vi "Serial Write to DB.vi"(8 "error in":errorcluster, 9 "Chamber ID":T2(array[cluster])=[{"Chamber name"="Analysis", "Trip pressure"=5e-07}, {"Chamber name"="Prep", "Trip pressure"=3e-05}], 10 "AML Cluster const":T1[](array[typedef]), 11 "Data.PG in":refnum<class "LV-Data.PGSQL.lvclass">) -> (0 "error out":errorcluster, 1 "Paths":string[](array[string]), 2 "Successful Writes":bool[](array[boolean]), 3 "Data.PG out":refnum<class "LV-Data.PGSQL.lvclass">)   [LabVIEW 2019, in "PGC2D.lvlib"]
uses:
  PGC2D.lvlib
  <userlib>/LevyLab/LV-Data/LV-Data.PG/LV-Data.PGSQL.lvclass
  sandbox/Instrument.AML.GetAll--Cluster.ctl
  <userlib>/LevyLab/LV-Data/LV-Data.PG/API/Write Variable (one-row).vi
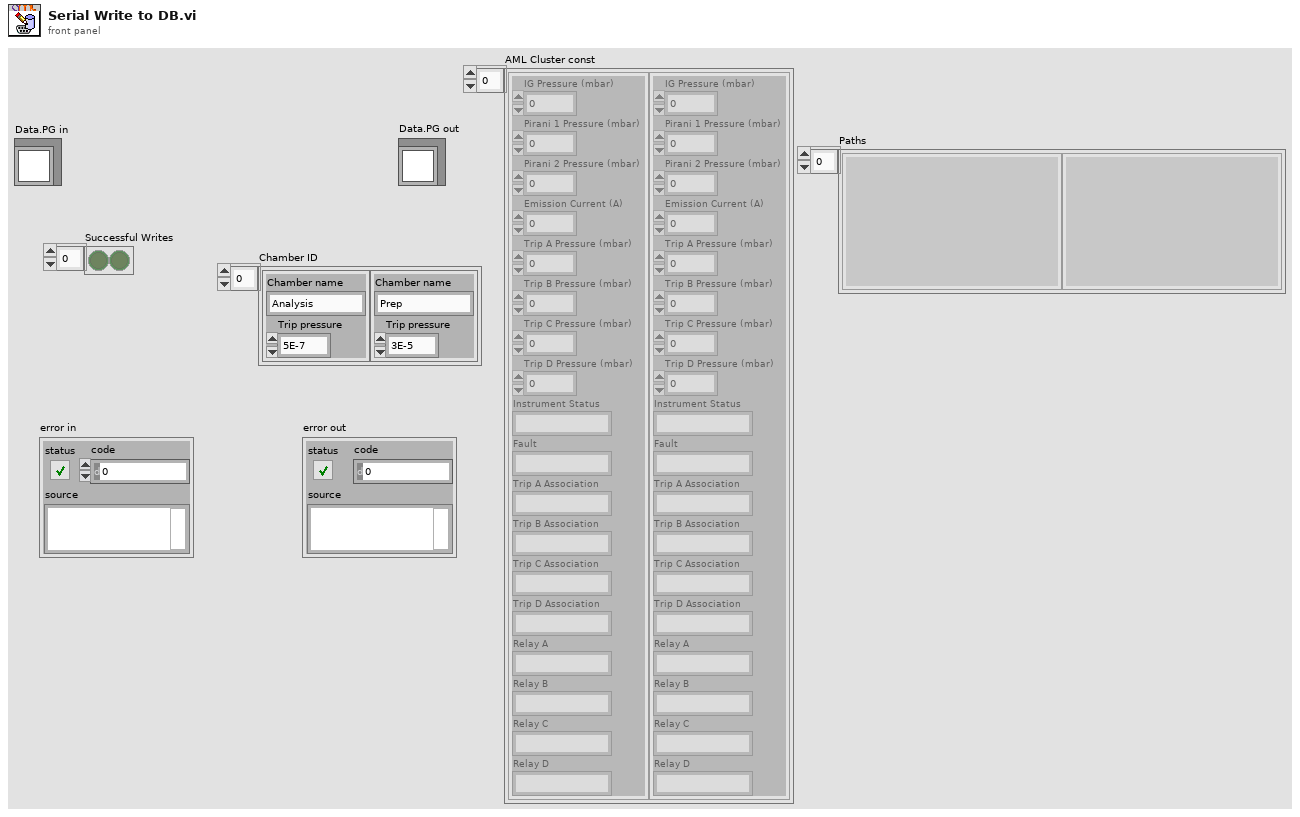
[diagram p1: front panel]
types:
  T1 = typedef "Instrument.AML.GetAll--Cluster.ctl" = cluster{"IG Pressure (mbar)":dbl, "Pirani 1 Pressure (mbar)":dbl, "Pirani 2 Pressure (mbar)":dbl, "Emission Current (A)":dbl, "Trip A Pressure (mbar)":dbl, "Trip B Pressure (mbar)":dbl, "Trip C Pressure (mbar)":dbl, "Trip D Pressure (mbar)":dbl, "Instrument Status":string, "Fault":string, "Trip A Association":string, "Trip B Association":string, "Trip C Association":string, "Trip D Association":string, "Relay A":string, "Relay B":string, "Relay C":string, "Relay D":string}
  T2 = cluster{"Chamber name":string, "Trip pressure":dbl}[]
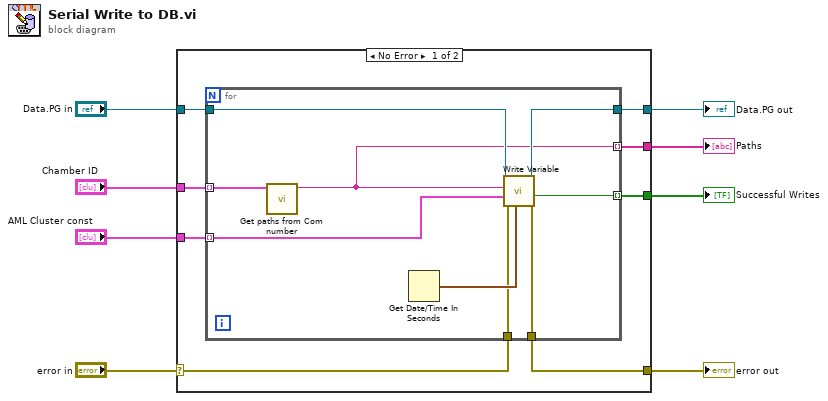
[diagram p0: block diagram]
diagram:
  n1 = case shown="No Error" "error in" {
    selector: "error in" -> [w16 w27]
    tunnel: [w15 w27] -> w7
    tunnel: "Data.PG in" -> [w14 w26]
    tunnel: [w13 w26] -> w5
    tunnel: [w12 _] -> w4
    tunnel: "AML Cluster const" -> [w11 _]
    tunnel: "Chamber ID" -> [w10 _]
    tunnel: [w9 _] -> w1
    frame No Error {
      n2 = for {
        tunnel: w16 -> [w24]
        tunnel: [w23] -> w15
        tunnel: w14 -> [w22]
        tunnel: [w21] -> w13
        tunnel: [w20] -> w12 mode=indexing
        tunnel: w11 -> [w19] mode=indexing
        tunnel: w10 -> [w17] mode=indexing
        tunnel: [w18] -> w9 mode=indexing
        n3 = call "Get paths from Com number.vi"("Chamber ID"=w17) -> ("paths"=w18:string)  [unwired: 10 in]
        n4 = Get Date/Time In Seconds() -> (seconds since 1Jan1904=w25:timestamp)
        n5 = call-poly <userlib>:"Write Variable.vi"("Time Stamp"=w25, "error in (no error)"=w24, "Data"=w19, "variable"=w18, "Data.PG in"=w22) -> ("error out"=w23:errorcluster, "Wrote to DB?"=w20:bool, "Data.PG out"=w21:refnum<class "LV-Data.PGSQL.lvclass">)  [unwired: 3 in, 1 out]
      }
    }
    frame Error {
    }
  }
  "error out" <- w7
  "Data.PG out" <- w5
  "Successful Writes" <- w4
  "Paths" <- w1
